vi "Updater Uninstall CrypKey.vi"(8 "error in (no error)":errorcluster, 11 "Spartan Install Path":path) -> (0 "error out":errorcluster)   [LabVIEW 2011]
uses:
  <vilib>/registry/registry.llb/Read Registry Value Simple STR.vi
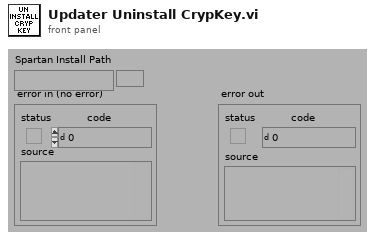
[diagram p1: front panel]
types:
  T1 = typedef "Registry refnum.ctl" = refnum<k1>
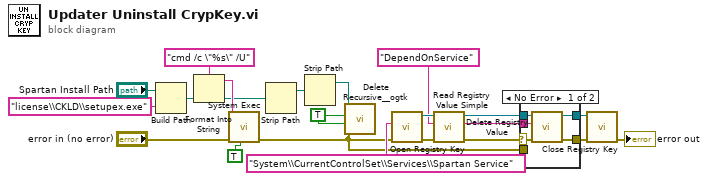
[diagram p0: block diagram]
diagram:
  w1 = "DependOnService" ("subkey")
  w11 = TRUE ("Recursive? (FALSE)")
  n1 = Build Path(base path="Spartan Install Path", name or relative path="license\\CKLD\\setupex.exe") -> (appended path=w14:path)
  n2 = Format Into String(format string="cmd /c \"%s\" /U", w14) -> (resulting string=w15:string)  [unwired: 2 in, 1 out]
  n3 = call <vilib>:"System Exec.vi"("run minimized? (F)"=TRUE, "error in (no error)"="error in (no error)", "command line"=w15) -> ("error out"=w6:errorcluster)  [unwired: 5 in, 3 out]
  n4 = Strip Path(path=w14) -> (stripped path=w13:path)  [unwired: 1 out]
  n5 = Strip Path(path=w13) -> (stripped path=w12:path)  [unwired: 1 out]
  n6 = call "Delete Recursive__ogtk.vi"("error in (no error)"=w6, "Ignore Read-Only? (FALSE)"=w11, "Recursive? (FALSE)"=w11, "Path"=w12) -> ()  [unwired: 6 in, 2 out]
  n7 = call <vilib>:"Open Registry Key.vi"("error in (no error)"=w6, "subkey"="System\\CurrentControlSet\\Services\\Spartan Service") -> ("error out"=w5:errorcluster, "refnum out"=w4:T1)  [unwired: 8 in]
  n8 = call-poly <vilib>:"Read Registry Value Simple.vi"("error in (no error)"=w5, "value"=w1, "refnum"=w4) -> ("error out"=w2:errorcluster, "refnum out"=w3:T1)  [unwired: 3 in, 2 out]
  n9 = case shown="No Error" w2 {
    selector: w2 -> [w24 _]
    tunnel: [w25 w27] -> w10
    tunnel: w6 -> [_ w27]
    tunnel: w3 -> [w23 w26]
    tunnel: [w22 w26] -> w7
    tunnel: w1 -> [w21 _]
    frame No Error {
      n10 = call <vilib>:"Delete Registry Value.vi"("error in (no error)"=w24, "value"=w21, "refnum"=w23) -> ("error out"=w25:errorcluster, "refnum out"=w22:T1)  [unwired: 7 in]
    }
    frame Error {
    }
  }
  n11 = call <vilib>:"Close Registry Key.vi"("error in (no error)"=w10, "refnum"=w7) -> ("error out"=→"error out":errorcluster)  [unwired: 5 in]
